vi "Boradcat All Notifier.vi"(7 "Timeout":i32=-1, 8 "error in (no error)":errorcluster, 10 "Notification In":variant, 11 "Notifier Controller in":refnum<class "Notifier Controller.lvclass">) -> (0 "error out":errorcluster, 3 "Notifier Controller out":refnum<class "Notifier Controller.lvclass">)   [LabVIEW 2022 SP3, in "Notifier Controller.lvclass"]
uses:
  Notifier Controller.lvclass
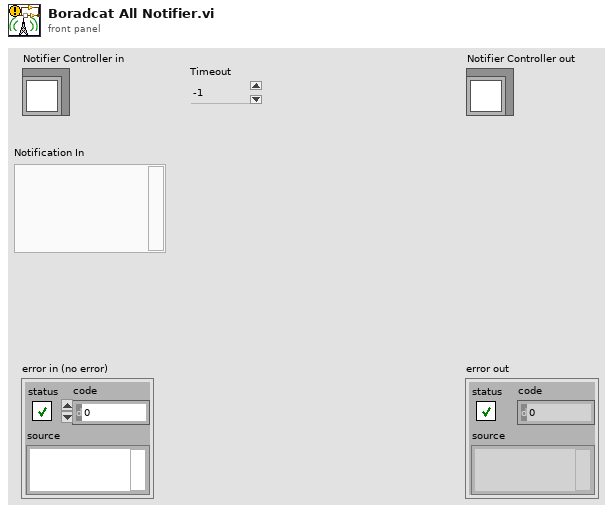
[diagram p1: front panel]
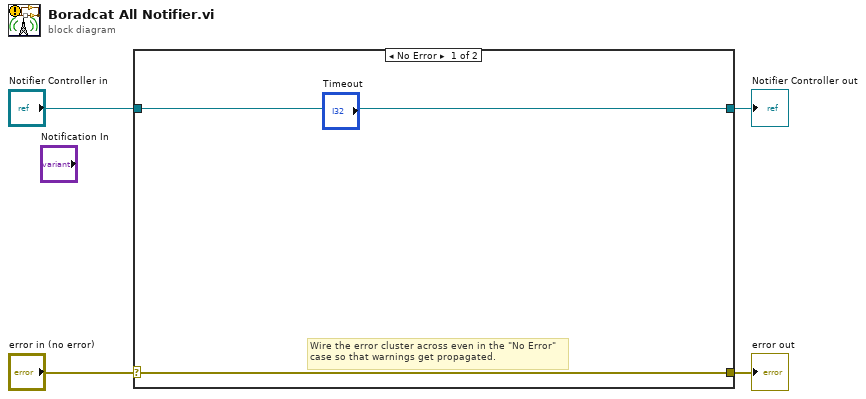
[diagram p0: block diagram]
diagram:
  n1 = case shown="No Error" "error in (no error)" {
    selector: "error in (no error)" -> [w5 w8]
    tunnel: [w5 w8] -> w3
    tunnel: [w6 w7] -> w1
    tunnel: "Notifier Controller in" -> [w6 w7]
    frame No Error {
      # "Wire the error cluster across even in the \"No Error\"\ncase so that warnings get propagated."
    }
    frame Error {
    }
  }
  "error out" <- w3
  "Notifier Controller out" <- w1
